vi "PH_Sixpack.GetUnitInformation.vi"(0 "i ref in":refnum<vi>, 4 "Device Error in":errorcluster, 5 "error in (no error)":errorcluster) -> (13 "Temperature / °C":i16, 14 "i ref out":refnum<vi>, 15 "FirmawareVersion":u8, 16 "Serial Number":u16, 17 "RESETFLAG":bool, 18 "Device Error out":errorcluster, 19 "error out":errorcluster)   [LabVIEW 2014, in "PH_Sixpack.lvlib"]
doc: "This VI queries the current instrument firmware revision and instrument driver revision.\nThis Instrument Driver's Revision number is 1.0 and is compatible with Instrument Firmware Revision 1.6.2\n(Instrument Driver Name)\nCreated By: Jupitec GmbH\nRelease Date:Feb 2002\nOriginally Developed in LabVIEW Version:\nModification History: \nNone"
uses:
  PH_Sixpack.lvlib
  instr.lib/SixPack/Sixpack - Driver.lvlib
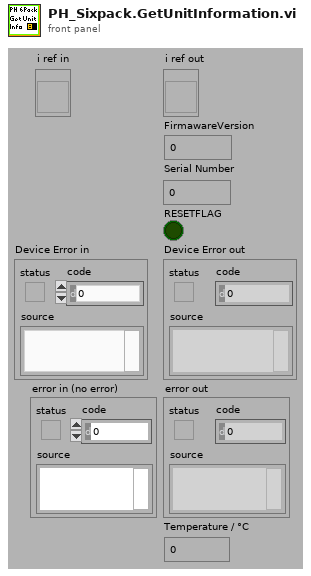
[diagram p1: front panel]
types:
  T1 = typedef "PH_Sixpack.lvlib/PH_Sixpack.i attribute.ctl" = cluster{"Information":cluster{"SixPack ID(0)":u16, "BaudRate(19200)":u16, "COM Port":enum32{"COM1", "COM2", "COM3", "COM4", "COM5", "COM6", "COM7", "COM8", "COM9"}, "HANDLE":i32}, "Serial Number":dbl, "Firmwareversion":dbl, "Axes":T2[], "Status":T14, "Axis to do a RefSearch":i32, "GUI Refs":cluster{"Information":refnum<vi>, "Serial Number":refnum<vi>, "Firmwareversion":refnum<vi>, "Status":refnum<vi>, "Axis to do a RefSearch":refnum<vi>, "Axes Configuration (Sixpack)":refnum<vi>, "Inputs":refnum<vi>, "PeriodicInterval [ms]":refnum<vi>}, "Constructor finished":bool, "Ignore Error":bool}
  T2 = typedef "PH_Sixpack.lvlib/PH_Sixpack.Axis Cluster.ctl" = cluster{"Config":T3, "To set?":cluster{"VmaxAmax":bool, "I max":bool, "VStartVminDivi":bool, "Ref Search Parameter":bool, "Stopswitch Limits":bool, "Axis Parameter":bool, "I Control":bool}}
  T3 = typedef "PH_Sixpack.lvlib/PH_Sixpack.Axis Configuration.ctl" = cluster{"VmaxAmax":T4, "I max (50%)":T5, "VStartVminDivi":T6, "Ref Search Parameter":T7, "Stopswitch Limits":T8, "Axis Parameter":T9, "I Control":T12}
  T4 = typedef "Sixpack - Driver.lvlib/VmaxAmax.ctl" = cluster{"VMax(511)":u16, "AMax(128)":u16}
  T5 = typedef "Sixpack - Driver.lvlib/PeakCurrent.ctl" = dbl
  T6 = typedef "Sixpack - Driver.lvlib/VStartVmin.ctl" = cluster{"VStart(5)":u16, "Vmin(4)":u16, "Div i (2)":enum8{"0", "1", "2", "3"}}
  T7 = typedef "Sixpack - Driver.lvlib/Ref Search Parameter.ctl" = cluster{"VRefMax(100)":u16, "DebouncingTime (22ms)":u8}
  T8 = typedef "Sixpack - Driver.lvlib/Stopswitch Limits.ctl" = cluster{"MinLeft(0)":u16, "MaxRight(1023)":u16}
  T9 = typedef "Sixpack - Driver.lvlib/Motor Parameter.ctl" = cluster{"Poslimit (6400)":u32, "P5 Bits":T10, "P6 Bits":T11}
  T10 = typedef "Sixpack - Driver.lvlib/MotorParameter_P5.ctl" = cluster{"MT_PI":bool, "MT_ROTARY":bool, "MT_AUTONULLCMD":bool, "MT_TESTNULL":bool, "MT_NULLLEFT":bool, "MT_NULLCENTRE":bool, "MT_STOPNULL":bool, "MT_FILTERSWITCH":bool}
  T11 = typedef "Sixpack - Driver.lvlib/MotorParameter_P6.ctl" = cluster{"MT_OPTIMIZEWAY":bool, "MT_FASTREF":bool, "MT_MECHREF":bool, "MT_DELAYTESTNULL":bool, "MT_STOPSOFT":bool, "MT_STOPNOREF":bool, "MT_NULLPOSITIVE":bool, "MUT_STOPFULSTEPS":bool}
  T12 = typedef "Sixpack - Driver.lvlib/Current Control.ctl" = cluster{"PowerDownDelay (500)":u16, "PowerDown (0%)":T13, "Standing (50%)":T13, "Running (75%)":T13, "Accelerating (100%)":T13}
  T13 = typedef "Sixpack - Driver.lvlib/Current.ctl" = enum8{"100%", "75%", "50%", "38%", "25%", "19%", "13%", "9%", "0%"}
  T14 = typedef "PH_Sixpack.lvlib/PH_Sixpack.Status.ctl" = enum32{"None", "Init", "Configure", "configured", "Close", "closed"}
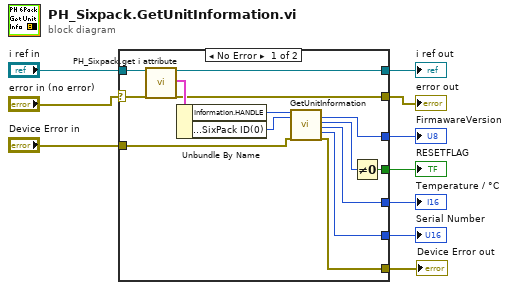
[diagram p0: block diagram]
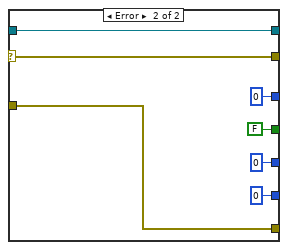
[diagram p2: hidden frame]
diagram:
  n1 = case shown="No Error" "error in (no error)" {
    selector: "error in (no error)" -> [w11 w30]
    tunnel: "i ref in" -> [w24 w31]
    tunnel: [w22 u16 0 ("SerialNumber")] -> w9
    tunnel: [w21 i16 0 ("Temperature")] -> w8
    tunnel: [w20 FALSE] -> w7
    tunnel: [w19 u8 0 ("FirmwareRevision")] -> w6
    tunnel: [w15 w31] -> w5
    tunnel: [w14 w30] -> w4
    tunnel: "Device Error in" -> [w13 w29]
    tunnel: [w12 w29] -> w2
    frame No Error {
      n2 = call "PH_Sixpack.get i attribute.vi"("i ref in"=w24, "error in (no error)"=w11) -> ("i ref out"=w15:refnum<vi>, "i attribute"=w23:T1, "error out"=w14:errorcluster)  [unwired: 15 in]
      n3 = Unbundle By Name(w23) -> ("Information.HANDLE"=w17:i32, "Information.SixPack ID(0)"=w18:u16)
      n4 = call "GetUnitInformation.vi"("handle in"=w17, "UnitAddress(0)"=w18, "error in"=w13) -> ("FirmwareRevision"=w19:u8, "ResetFlag"=w16:u8, "Temperature"=w21:i16, "SerialNumber"=w22:u16, "error out"=w12:errorcluster)  [unwired: 11 in, 1 out]
      n5 = Not Equal To 0?(x=w16) -> (x != 0?=w20:bool)
    }
    frame Error {
    }
  }
  "error out" <- w4
  "i ref out" <- w5
  "Temperature / °C" <- w8
  "Serial Number" <- w9
  "RESETFLAG" <- w7
  "FirmawareVersion" <- w6
  "Device Error out" <- w2
